vi "Comparison By Year Born.vi"(10 "Person B":T1={"ID"=0, "Family Name"="Doe", "Given Name"="John", "Birth Date"=timestamp(3533142714.9178333 s since 1904-01-01)} {"Birth Date" format="%<%Y/%b/%d>T"}, 11 "Person A":T1={"ID"=0, "Family Name"="Smith", "Given Name"="John", "Birth Date"=timestamp(3533056306.0488334 s since 1904-01-01)} {"Birth Date" format="%<%Y/%b/%d>T"}) -> (3 "Swap?":bool)   [LabVIEW 2023]
doc: "This VI says that the two values should swap if Person A has a later birthday. If they have the same birthday, then they should swap if Person A has an alphabetically later name than Person B, checking last name first and then first name."
uses:
  Person Information.ctl
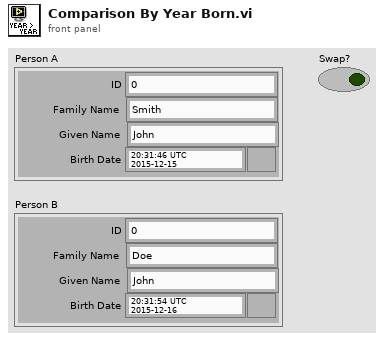
[diagram p1: front panel]
types:
  T1 = typedef "Person Information.ctl" = cluster{"ID":u32, "Family Name":string, "Given Name":string, "Birth Date":timestamp}
  T2 = typedef "LVDateTimeRec.ctl" = cluster{"fractional second":dbl, "second":i32, "minute":i32, "hour":i32, "day of month":i32, "month":i32, "year":i32, "day of week":i32, "day of year":i32, "DST":i32}
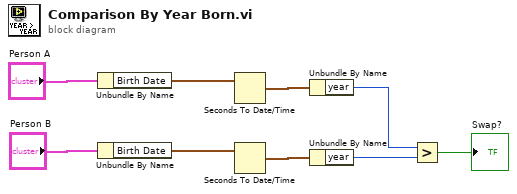
[diagram p0: block diagram]
diagram:
  n1 = Unbundle By Name("Person A") -> ("Birth Date"=w7:timestamp)
  n2 = Unbundle By Name("Person B") -> ("Birth Date"=w6:timestamp)
  n3 = Seconds To Date/Time(time stamp (now)=w7) -> (date time rec=w4:T2)  [unwired: 1 in]
  n4 = Seconds To Date/Time(time stamp (now)=w6) -> (date time rec=w5:T2)  [unwired: 1 in]
  n5 = Unbundle By Name(w4) -> ("year"=w3:i32)
  n6 = Unbundle By Name(w5) -> ("year"=w2:i32)
  n7 = Greater?(x=w3, y=w2) -> (0:→"Swap?":bool)
